vi "Array and Dbl to 1 results.vi"(2 "Result3":dbl=nan, 3 "Result 1 Array":dbl[](array[numeric]), 4 "Result 3 Array":dbl[](array[numeric]), 5 "Result2":dbl=nan, 6 "Result 2 Array":dbl[](array[numeric]), 7 "Result1":dbl) -> (0 "Length":i32[](array[numeric]), 1 "Array Set":dbl[][](array[numeric]))   [LabVIEW 2017]
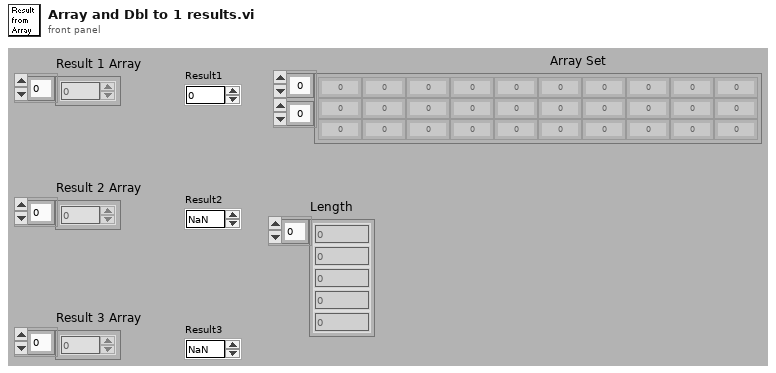
[diagram p1: front panel]
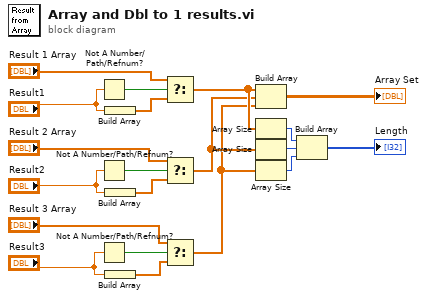
[diagram p0: block diagram]
diagram:
  n1 = Not A Number/Path/Refnum?(number/path/refnum="Result1") -> (NaN/Path/Refnum?=w6:bool)
  n2 = Not A Number/Path/Refnum?(number/path/refnum="Result2") -> (NaN/Path/Refnum?=w4:bool)
  n3 = Not A Number/Path/Refnum?(number/path/refnum="Result3") -> (NaN/Path/Refnum?=w5:bool)
  n4 = Build Array("Result1") -> (w12:dbl[])
  n5 = Build Array("Result2") -> (w10:dbl[])
  n6 = Build Array("Result3") -> (w11:dbl[])
  n7 = Select(t="Result 1 Array", s=w6, f=w12) -> (s? t:f=w3:dbl[])
  n8 = Select(t="Result 2 Array", s=w4, f=w10) -> (s? t:f=w2:dbl[])
  n9 = Select(t="Result 3 Array", s=w5, f=w11) -> (s? t:f=w1:dbl[])
  n10 = Build Array(w3, w2, w1) -> (→"Array Set":dbl[][])
  n11 = Array Size(array=w3) -> (size(s)=w15:i32)
  n12 = Array Size(array=w2) -> (size(s)=w16:i32)
  n13 = Array Size(array=w1) -> (size(s)=w17:i32)
  n14 = Build Array(w15, w16, w17) -> (→"Length":i32[])
